vi "BoolToU16.vi"(11 "Boolean":bool=TRUE) -> (3 "Numeric":u16)   [LabVIEW 2012]
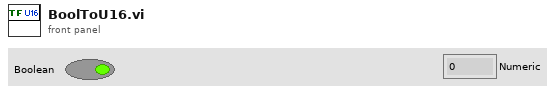
[diagram p1: front panel]
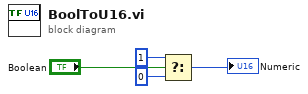
[diagram p0: block diagram]
diagram:
  n1 = Select(t=u16 1, s="Boolean", f=u16 0) -> (s? t:f=→"Numeric":u16)
